vi "Get Motor Velocity Setpoints.vi"(8 "error in (no error)":errorcluster, 11 "motor communication in":refnum<class "NI_Robotics_Motor Communication.lvclass">[](array[class])) -> (0 "error out":errorcluster, 1 "failed?":bool[](array[boolean]), 2 "velocities":dbl[](array[numeric]), 3 "motor communication out":refnum<class "NI_Robotics_Motor Communication.lvclass">[](array[class]))   [LabVIEW 2017, in "NI_Robotics_Motor Communication.lvclass"]
doc: "Returns the angles or angular velocity setpoints from the motor communication session. You must manually select the polymorphic instance to use."
uses:
  <vilib>/robotics/Actuation/Motor Communication/NI_Robotics_Motor Communication.lvclass
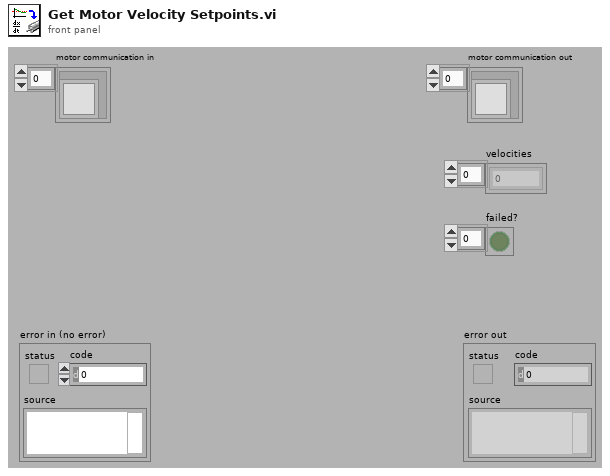
[diagram p1: front panel]
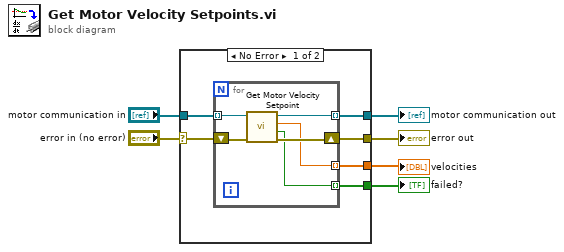
[diagram p0: block diagram]
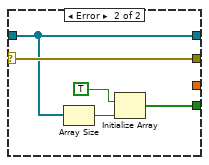
[diagram p2: hidden frame]
diagram:
  n1 = case shown="No Error" "error in (no error)" {
    selector: "error in (no error)" -> [w7 w23]
    tunnel: [w8 w23] -> w5
    tunnel: "motor communication in" -> [w12 w19]
    tunnel: [w11 w19] -> w3
    tunnel: [w10 _] -> w2
    tunnel: [w9 w20] -> w1
    frame No Error {
      n2 = for {
        tunnel: w12 -> [w18] mode=indexing
        tunnel: [w17] -> w11 mode=indexing
        shift-right: [w16] -> w8
        shift-left: w7 -> [w15]
        tunnel: [w14] -> w10 mode=indexing
        tunnel: [w13] -> w9 mode=indexing
        n3 = call <vilib>:"Get Motor Velocity Setpoint.vi"("error in (no error)"=w15, "motor communication in"=w18) -> ("error out"=w16:errorcluster, "failed?"=w13:bool, "velocity"=w14:dbl, "motor communication out"=w17:refnum<class "NI_Robotics_Motor Communication.lvclass">)  [unwired: 6 in]
      }
    }
    frame Error {
      n4 = Array Size(array=w19) -> (size(s)=w21:i32)
      n5 = Initialize Array(TRUE, w21) -> (w20:bool[])
    }
  }
  "error out" <- w5
  "motor communication out" <- w3
  "velocities" <- w2
  "failed?" <- w1
